vi "Teleop.vi"(10 "Match Info":T1={"Autonomous Elapsed Seconds"=0.0, "TeleOp Elapsed Seconds"=0.0, "Disabled Elapsed Seconds"=0.0, "Visited Autonomous"=FALSE, "Visited TeleOp"=FALSE, "Visited Disabled"=FALSE, "Autonomous Settings"={"Autonomous Style"=enum."Independent", "VI Refnum"=refnum}}, 11 "Call Context":T2) -> ()   [LabVIEW 2014]
doc: "This VI is called for each TeleOp packet received from the DS where the robot is not disabled. It is often used to read from the joysticks and update I/O or to update setpoints for timed control loops. It should complete and return within 20 milliseconds or it may miss DS packets."
uses:
  <vilib>/Rock Robotics/WPI/DriverStation/WPI_DriverStationDerivedRobotMode.ctl
  <vilib>/Rock Robotics/WPI/DriverStation/WPI_DriverStationMatch Info.ctl
  <vilib>/Rock Robotics/WPI/RobotDrive/WPI_RobotDriveGetSetRefNum.vi
  <vilib>/Rock Robotics/WPI/Joystick/WPI_JoystickGetSetRefNum.vi
  Robot Global Data.vi
panel:
  out "Sample Slider 0":dbl(slide) scale=0.0..5.0
  out "Sample Boolean 1":bool
  out "Sample Boolean 0":bool
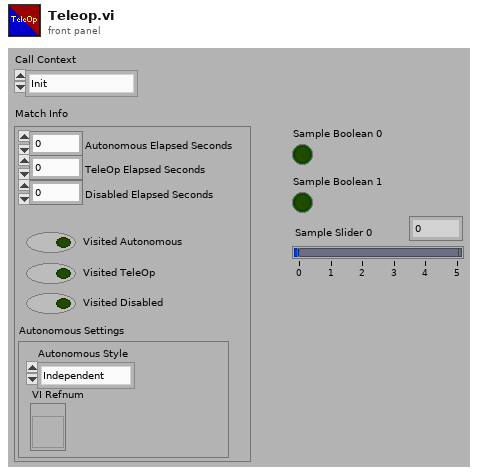
[diagram p1: front panel]
types:
  T1 = typedef "WPI_DriverStationMatch Info.ctl" = cluster{"Autonomous Elapsed Seconds":dbl, "TeleOp Elapsed Seconds":dbl, "Disabled Elapsed Seconds":dbl, "Visited Autonomous":bool, "Visited TeleOp":bool, "Visited Disabled":bool, "Autonomous Settings":cluster{"Autonomous Style":enum16{"Iterative", "Independent"}, "VI Refnum":refnum<vi>}}
  T2 = typedef "WPI_DriverStationDerivedRobotMode.ctl" = enum16{"Init", "Execute", "Stop"}
  T3 = typedef "WPI_RobotDriveDevRef.ctl" = cluster{"DevStatus":errorcluster, "Motors[]":T4[], "Square Inputs":bool, "Max Output":dbl}
  T4 = typedef "WPI_MotorControlDeviceRef.ctl" = cluster{"DeviceStatus":errorcluster, "Type":enum16{"PWM", "CAN"}, "PWM":cluster{"Digital Module":T5, "PWM Channel":T6, "DeadBand":T7}, "CAN":cluster{"Device Number":u8, "Control Mode":T8, "Semaphore":T9, "Max Vout":dbl}, "Invert":bool, "TransformRef":T10, "InvTransformRef":T10}
  T5 = typedef "FPGA_TypedefDigitalModule.ctl" = enum16{"Digital Module 1", "Digital Module 2"}
  T6 = typedef "FPGA_DIOPWMChannel.ctl" = enum8{"PWM 1", "PWM 2", "PWM 3", "PWM 4", "PWM 5", "PWM 6", "PWM 7", "PWM 8", "PWM 9", "PWM 10", "Invalid"}
  T7 = typedef "WPI_PWMDeadband.ctl" = cluster{"Name":string, "maxPositivePwm":i32, "minPositivePwm":i32, "centerPwm":i32, "maxNegativePwm":i32, "minNegativePwm":i32, "angularRange":u16}
  T8 = typedef "WPI_CANJaguar_ControlMode.ctl" = enum8{"Percent VBus", "Current", "Speed", "Position", "Voltage"}
  T9 = typedef "Semaphore RefNum" = refnum<k1>
  T10 = typedef "WPI_PWMTransform_ConPane.ctl" = refnum<vi>
  T11 = typedef "WPI_JoystickDevRef.ctl" = cluster{"Device":T12}
  T12 = typedef "WPI_JoystickDeviceEnum.ctl" = enum16{"USB 0", "USB 1", "USB 2", "USB 3", "USB 4", "USB 5"}
  T13 = cluster{"Button 1":bool, "Button 2":bool, "Button 3":bool, "Button 4":bool, "Button 5":bool, "Button 6":bool, "Button 7":bool, "Button 8":bool, "Button 9":bool, "Button 10":bool, "Button 11":bool, "Button 12":bool}
  T14 = cluster{"axis 1 (x)":dbl, "axis 2 (y)":dbl, "axis 3 (throttle)":dbl, "axis 4":dbl, "axis 5":dbl, "axis 6":dbl}
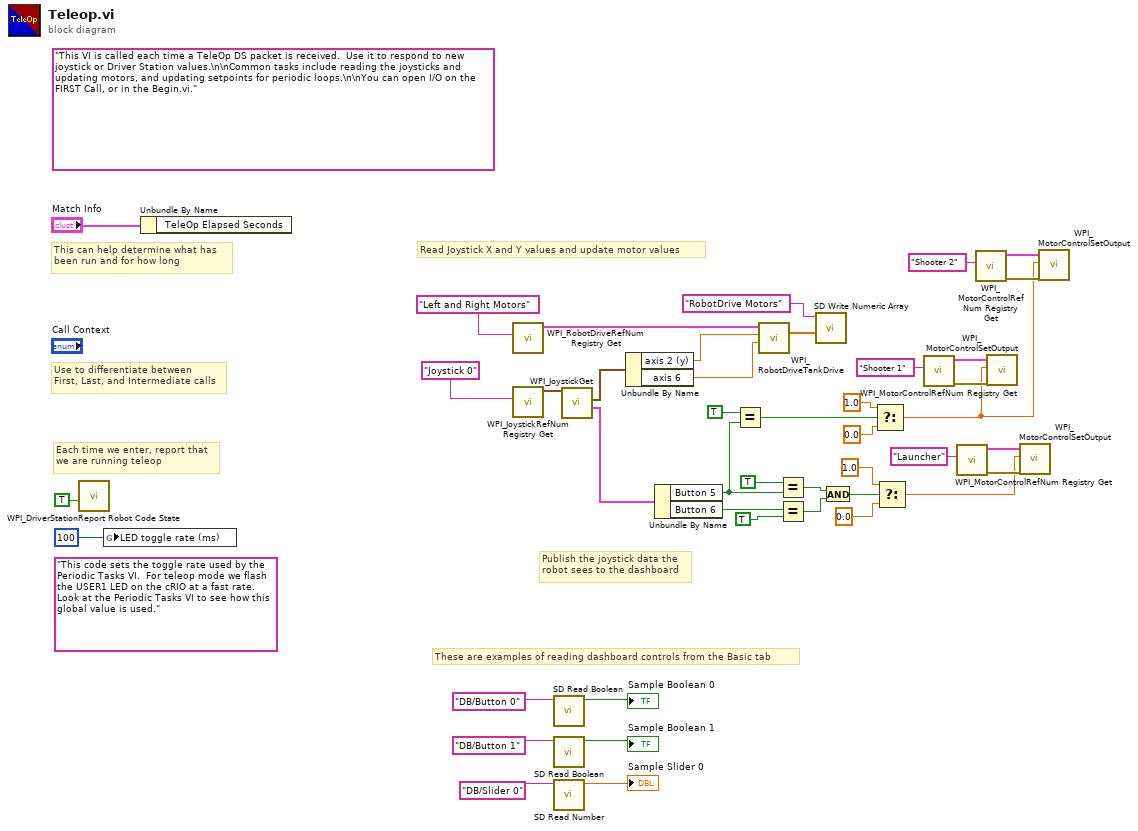
[diagram p0: block diagram]
diagram:
  (unwired) "This code sets the toggle rate used by the Periodic Tasks VI.  For teleop mode we flash the USER1 LED on the cRIO at a fast rate.  Look at the Periodic Tasks VI to see how this global value is used."
  (unwired) "This VI is called each time a TeleOp DS packet is received.  Use it to respond to new joystick or Driver Station values.\n\nCommon tasks include reading the joysticks and updating motors, and updating setpoints for periodic loops.\n\nYou can open I/O on the FIRST Call, or in the Begin.vi."
  # "These are examples of reading dashboard controls from the Basic tab"
  # "Publish the joystick data the\nrobot sees to the dashboard"
  # "Each time we enter, report that\nwe are running teleop"
  # "Use to differentiate between\nFirst, Last, and Intermediate calls"
  # "This can help determine what has\nbeen run and for how long"
  # "Read Joystick X and Y values and update motor values"
  n1 = call <vilib>:"WPI_DriverStationReport Robot Code State.vi"("TeleOp"=TRUE ("Autonomous")) -> ()  [unwired: 10 in, 1 out]
  n2 = global write "Robot Global Data.vi" "LED toggle rate (ms)"(u32 100 ("LED ms toggle rate")) -> ()
  n3 = Unbundle By Name("Match Info") -> ()  [unwired: 1 out]
  n4 = call <vilib>:"WPI_RobotDriveRefNum Registry Get.vi"("refnum name"="Left and Right Motors") -> ("RobotDriveDevRef"=w41:T3)  [unwired: 1 in, 9 out]
  n5 = call <vilib>:"WPI_JoystickRefNum Registry Get.vi"("refnum name"="Joystick 0") -> ("JoystickDevRef"=w16:T11)  [unwired: 1 in, 9 out]
  n6 = call <vilib>:"SD Read Boolean.vi"("Name"="DB/Button 0" ("refnum name")) -> ("Boolean"=→"Sample Boolean 0":bool)  [unwired: 8 in, 2 out]
  n7 = call <vilib>:"SD Read Boolean.vi"("Name"="DB/Button 1" ("refnum name")) -> ("Boolean"=→"Sample Boolean 1":bool)  [unwired: 8 in, 2 out]
  n8 = call <vilib>:"SD Read Number.vi"("Name"="DB/Slider 0" ("refnum name")) -> ("Numeric"=→"Sample Slider 0":dbl)  [unwired: 8 in, 2 out]
  n9 = call <vilib>:"WPI_JoystickGet.vi"("JoystickDevRef"=w16) -> ("Buttons"=w15:T13, "Axes"=w7:T14)  [unwired: 1 in, 4 out]
  n10 = Unbundle By Name(w7) -> ("axis 2 (y)"=w6:dbl, "axis 6"=w5:dbl)
  n11 = Unbundle By Name(w15) -> ("Button 5"=w20:bool, "Button 6"=w26:bool)
  n12 = Equal?(x=TRUE, y=w20) -> (x = y?=w17:bool)
  n13 = call <vilib>:"WPI_RobotDriveTankDrive.vi"("Right axis value"=w5, "Left axis value"=w6, "RobotDriveDevRef"=w41) -> ("Motor Values"=w36:dbl[])  [unwired: 6 in, 2 out]
  n14 = Equal?(x=TRUE, y=w20) -> (x = y?=w28:bool)
  n15 = Equal?(x=w26, y=TRUE) -> (x = y?=w25:bool)
  n16 = call <vilib>:"SD Write Numeric Array.vi"("Numeric Array"=w36, "Name"="RobotDrive Motors") -> ()  [unwired: 8 in, 2 out]
  n17 = And(x=w28, y=w25) -> (x .and. y?=w24:bool)
  n18 = Select(t=1.0 ("Output"), s=w17, f=0.0 ("Output")) -> (s? t:f=w1:dbl)
  n19 = Select(t=1.0 ("Output"), s=w24, f=0.0 ("Output")) -> (s? t:f=w8:dbl)
  n20 = call <vilib>:"WPI_MotorControlRefNum Registry Get.vi"("refnum name"="Shooter 1") -> ("error out"=w13:errorcluster, "MotorControlDevRef"=w14:T4)  [unwired: 9 in]
  n21 = call <vilib>:"WPI_MotorControlRefNum Registry Get.vi"("refnum name"="Launcher") -> ("error out"=w10:errorcluster, "MotorControlDevRef"=w11:T4)  [unwired: 9 in]
  n22 = call <vilib>:"WPI_MotorControlRefNum Registry Get.vi"("refnum name"="Shooter 2") -> ("error out"=w3:errorcluster, "MotorControlDevRef"=w4:T4)  [unwired: 9 in]
  n23 = call <vilib>:"WPI_MotorControlSetOutput.vi"("error in (no error)"=w13, "Output"=w1, "MotorControlDevRef"=w14) -> ()  [unwired: 6 in, 3 out]
  n24 = call <vilib>:"WPI_MotorControlSetOutput.vi"("error in (no error)"=w10, "Output"=w8, "MotorControlDevRef"=w11) -> ()  [unwired: 6 in, 3 out]
  n25 = call <vilib>:"WPI_MotorControlSetOutput.vi"("error in (no error)"=w3, "Output"=w1, "MotorControlDevRef"=w4) -> ()  [unwired: 6 in, 3 out]
